vi "Initialize-notifiers.vi"(8 "error in (no error)":errorcluster, 11 "UI ref. in":refnum<data-value>) -> (0 "error out":errorcluster, 3 "UI ref.":refnum<data-value>)   [LabVIEW 2013, in "CameraVision.lvlib" / "CV-UI.lvclass"]
uses:
  CV-UI.lvclass
  Settings-source.ctl
  Image-selector.ctl
  Camera-selector.ctl
  Main/Mapping/Mapping-characteristic.ctl
  Display-selector.ctl
  CV-UI.lvclass/CV-UI.ctl
  Main/Mapping/CV-Mapping.lvclass
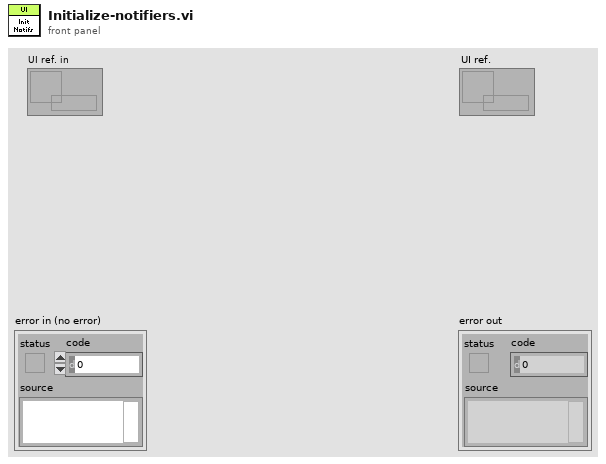
[diagram p1: front panel]
types:
  T1 = typedef "CameraVision.lvlib/CV-UI.lvclass/Display-selector.ctl" = enum32{"Single view", "Dual view", "Analysis", "History", "Temperature field", "Mapping", "Debug"}
  T2 = typedef "CameraVision.lvlib/CV-Mapping.lvclass/Mapping-characteristic.ctl" = enum16{"Average intensity [0-255]", "Peak intensity [0-255]", "Melt-pool size [mm²]", "Melt-pool aspect ratio []", "Melt-pool fragments []", "Average temperature [°C]", "Max. temperature [°C]", "Min. temperature [°C]", "Std. dev. temperature [°C]"}
  T3 = typedef "CameraVision.lvlib/CV-UI.lvclass/Camera-selector.ctl" = enum16{"Camera 1", "Camera 2"}
  T4 = typedef "CameraVision.lvlib/CV-UI.lvclass/Image-selector.ctl" = enum16{"Original", "Corrected", "Binary"}
  T5 = typedef "CameraVision.lvlib/CV-UI.lvclass/Settings-source.ctl" = enum16{"Custom", "Default", "Last used", "File"}
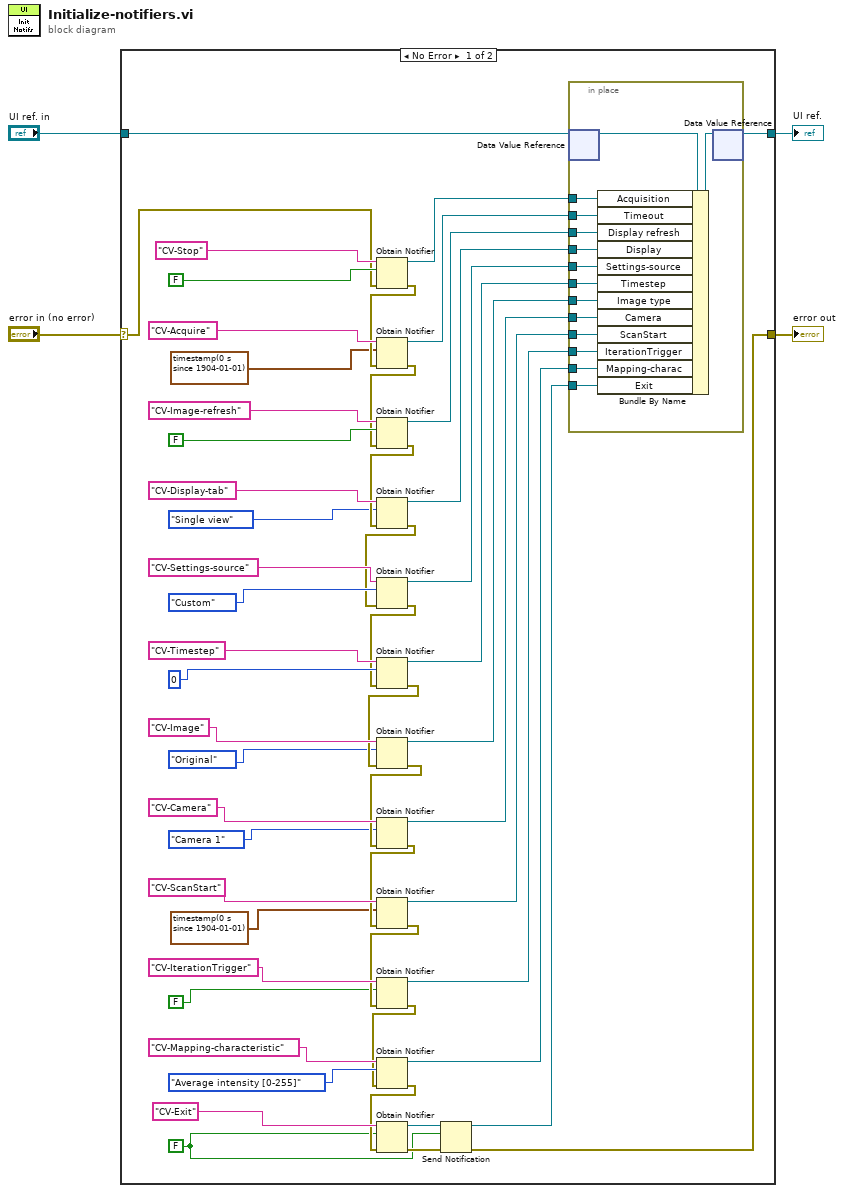
[diagram p0: block diagram]
diagram:
  n1 = case shown="No Error" "error in (no error)" {
    selector: "error in (no error)" -> [w9 w73]
    tunnel: [w6 w73] -> w3
    tunnel: "UI ref. in" -> [w57 w72]
    tunnel: [w56 w72] -> w1
    frame No Error {
      w5 = FALSE
      n2 = Obtain Notifier(name (unnamed)="CV-Stop", notification data type=FALSE, error in (no error)=w9) -> (notifier out=w10:refnum<notifier>, error out=w47:errorcluster)  [unwired: 1 in, 1 out]
      n3 = Obtain Notifier(name (unnamed)="CV-Acquire", notification data type=timestamp(0 s since 1904-01-01), error in (no error)=w47) -> (notifier out=w23:refnum<notifier>, error out=w48:errorcluster)  [unwired: 1 in, 1 out]
      n4 = Obtain Notifier(name (unnamed)="CV-Image-refresh", notification data type=FALSE, error in (no error)=w48) -> (notifier out=w22:refnum<notifier>, error out=w49:errorcluster)  [unwired: 1 in, 1 out]
      n5 = Obtain Notifier(name (unnamed)="CV-Display-tab", notification data type=Display-selector."Single view" ("Displays"), error in (no error)=w49) -> (notifier out=w21:refnum<notifier>, error out=w41:errorcluster)  [unwired: 1 in, 1 out]
      n6 = Obtain Notifier(name (unnamed)="CV-Settings-source", notification data type=Settings-source."Custom" ("Settings source"), error in (no error)=w41) -> (notifier out=w20:refnum<notifier>, error out=w42:errorcluster)  [unwired: 1 in, 1 out]
      n7 = Obtain Notifier(name (unnamed)="CV-Timestep", notification data type=0, error in (no error)=w42) -> (notifier out=w19:refnum<notifier>, error out=w39:errorcluster)  [unwired: 1 in, 1 out]
      n8 = Obtain Notifier(name (unnamed)="CV-Image", notification data type=Image-selector."Original" ("Image"), error in (no error)=w39) -> (notifier out=w18:refnum<notifier>, error out=w36:errorcluster)  [unwired: 1 in, 1 out]
      n9 = Obtain Notifier(name (unnamed)="CV-Camera", notification data type=Camera-selector."Camera 1" ("Camera selector"), error in (no error)=w36) -> (notifier out=w17:refnum<notifier>, error out=w32:errorcluster)  [unwired: 1 in, 1 out]
      n10 = Obtain Notifier(name (unnamed)="CV-ScanStart", notification data type=timestamp(0 s since 1904-01-01), error in (no error)=w32) -> (notifier out=w16:refnum<notifier>, error out=w26:errorcluster)  [unwired: 1 in, 1 out]
      n11 = Obtain Notifier(name (unnamed)="CV-IterationTrigger", notification data type=FALSE, error in (no error)=w26) -> (notifier out=w15:refnum<notifier>, error out=w25:errorcluster)  [unwired: 1 in, 1 out]
      n12 = Obtain Notifier(name (unnamed)="CV-Mapping-characteristic", notification data type=Mapping-characteristic."Average intensity [0-255]" ("Map characteristic"), error in (no error)=w25) -> (notifier out=w14:refnum<notifier>, error out=w12:errorcluster)  [unwired: 1 in, 1 out]
      n13 = Obtain Notifier(name (unnamed)="CV-Exit", notification data type=w5, error in (no error)=w12) -> (notifier out=w11:refnum<notifier>, error out=w7:errorcluster)  [unwired: 1 in, 1 out]
      n14 = Send Notification(notification=w5, notifier=w11, error in (no error)=w7) -> (notifier out=w8:refnum<notifier>, error out=w6:errorcluster)
      n15 = in-place {
        in-place-border: w10 -> [w58]
        in-place-border: w23 -> [w69]
        in-place-border: w22 -> [w68]
        in-place-border: w21 -> [w67]
        in-place-border: w20 -> [w66]
        in-place-border: w19 -> [w65]
        in-place-border: w18 -> [w64]
        in-place-border: w17 -> [w63]
        in-place-border: w16 -> [w62]
        in-place-border: w15 -> [w61]
        in-place-border: w14 -> [w60]
        in-place-border: w8 -> [w59]
        n16 = in-place-dvr #1(w57) -> (w71:refnum<class "CV-UI.lvclass">)  [unwired: 1 out]
        n17 = Bundle By Name(cluster=w71, "Acquisition"=w58, "Timeout"=w69, "Display refresh"=w68, "Display"=w67, "Settings-source"=w66, "Timestep"=w65, "Image type"=w64, "Camera"=w63, "ScanStart"=w62, "IterationTrigger"=w61, "Mapping-charac"=w60, "Exit"=w59) -> (w70:refnum<class "CV-UI.lvclass">)
        n18 = in-place-dvr #1(w70) -> (w56:refnum<data-value>)  [unwired: 1 out]
      }
    }
    frame Error {
    }
  }
  "error out" <- w3
  "UI ref." <- w1
